vi "dbl2i32.vi"() -> ()   [LabVIEW 2017]
panel:
  out "output array":dbl[](array[numeric])
  out "input array":dbl[](array[numeric])
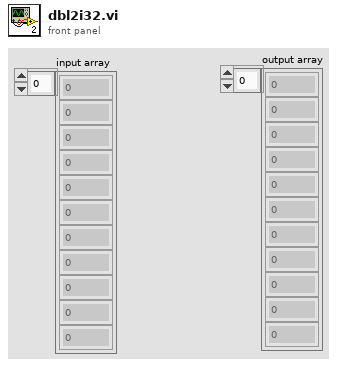
[diagram p1: front panel]
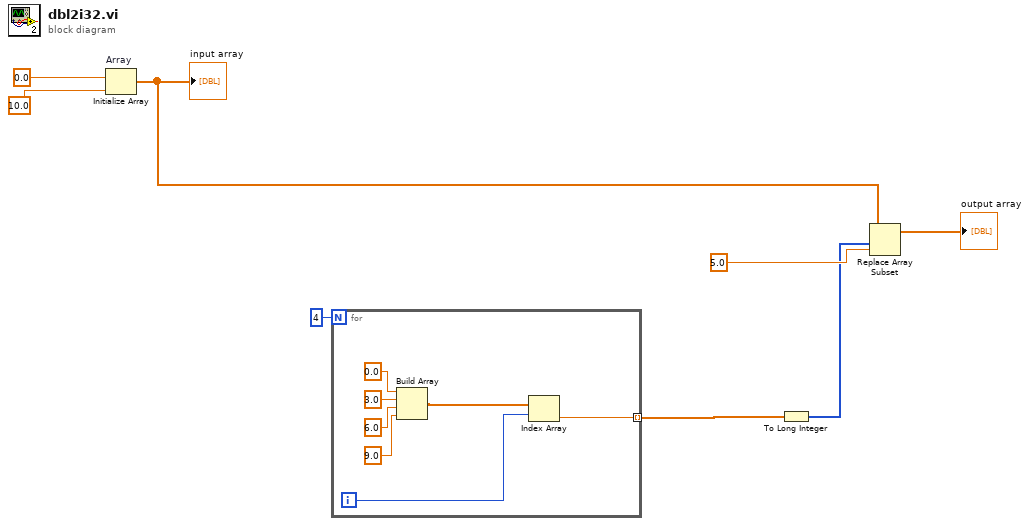
[diagram p0: block diagram]
diagram:
  n1 = Initialize Array "Array"(0.0 ("element"), 10.0 ("element")) -> (w6:dbl[])
  "input array" <- w6
  n2 = for {
    N: 4 -> [_]
    tunnel: [w9] -> w2 mode=indexing
    i -> [w10]
    n3 = Build Array(0.0 ("element"), 3.0 ("element"), 6.0 ("element"), 9.0 ("element")) -> (w11:dbl[])
    n4 = Index Array(array=w11, index=w10) -> (element=w9:dbl)
  }
  n5 = To Long Integer(number=w2) -> (32bit integer=w1:i32[])
  n6 = Replace Array Subset(array=w6, new element=5.0 ("element"), index=w1) -> (→"output array":dbl[])
